vi "Get Recoverable Network Streams Errors.vi"() -> (3 "recoverable network streams errors":i32[](array[numeric]))   [LabVIEW 2017]
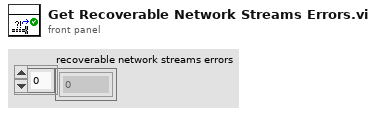
[diagram p1: front panel]
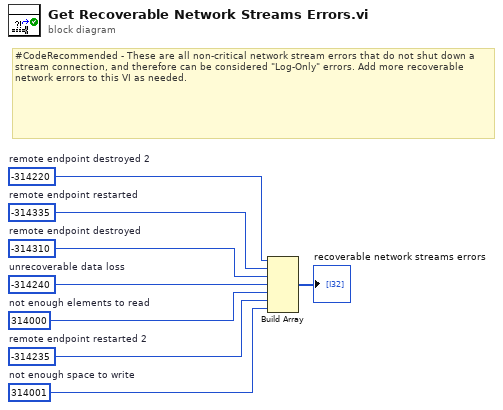
[diagram p0: block diagram]
diagram:
  w1 = -314220  # remote endpoint destroyed 2
  w3 = 314001  # not enough space to write
  w5 = 314000  # not enough elements to read
  w4 = -314235  # remote endpoint restarted 2
  w6 = -314240  # unrecoverable data loss
  w7 = -314310  # remote endpoint destroyed
  w8 = -314335  # remote endpoint restarted
  # "#CodeRecommended - These are all non-critical network stream errors that do not shut down a stream connection, and therefore can be considered \"Log-Only\" errors. Add more recoverable network errors to this VI as needed."
  n1 = Build Array(w1, w8, w7, w6, w5, w4, w3) -> (→"recoverable network streams errors":i32[])
